vi "Execute.vi"(8 "error in":errorcluster, 11 "Wait STEP in":refnum<class "Wait STEP.lvclass">) -> (0 "error out":errorcluster, 1 "Next Step?":bool, 2 "MSG":string, 3 "Wait STEP out":refnum<class "Wait STEP.lvclass">)   [LabVIEW 2014, in "Wait STEP.lvclass"]
uses:
  Wait STEP.lvclass
  reusable/Sequence/STEPS/STEP.lvclass/STEP.ctl
  reusable/Sequence/STEPS/LEAVES/Double/Switch DBL.lvclass/Switch DBL.ctl
  reusable/Sequence/STEPS/Write First Call.vi
  reusable/Sequence/STEPS/Read First Call.vi
  reusable/Sequence/STEPS/LEAVES/Double/Read val.vi
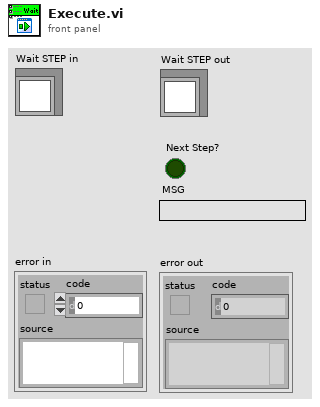
[diagram p1: front panel]
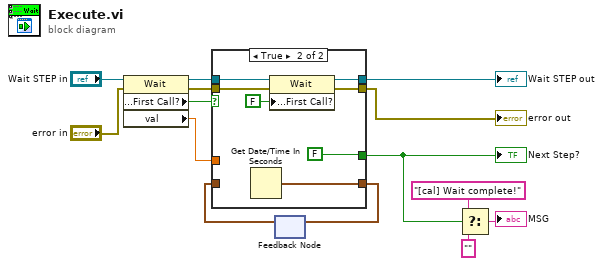
[diagram p0: block diagram]
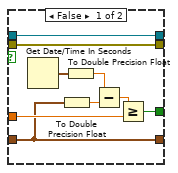
[diagram p2: hidden frame]
diagram:
  n1 = property class="Wait"(reference="Wait STEP in", error in="error in") -> (reference out=w12:refnum<class "Wait STEP.lvclass">, error out=w7:errorcluster, "Accessors:First Call?"=w13:bool, "val"=w10:dbl)
  n2 = feedback #1() -> (w11:timestamp)  [unwired: 1 in]
  n3 = case shown="True" w13 {
    tunnel: w12 -> [w20 w30]
    tunnel: [w16 w28] -> w1
    tunnel: w11 -> [w16 _]
    tunnel: w10 -> [w22 _]
    tunnel: [w21 FALSE] -> w5
    tunnel: [w20 w26] -> w9
    tunnel: w7 -> [w19 w25]
    tunnel: [w19 w24] -> w6
    frame False {
      n4 = Get Date/Time In Seconds() -> (seconds since 1Jan1904=w18:timestamp)
      n5 = To Double Precision Float(number=w16) -> (double precision float=w15:dbl)
      n6 = To Double Precision Float(number=w18) -> (double precision float=w17:dbl)
      n7 = Subtract(x=w17, y=w15) -> (x-y=w23:dbl)
      n8 = Greater Or Equal?(x=w23, y=w22) -> (x >= y?=w21:bool)
    }
    frame True {
      n9 = Get Date/Time In Seconds() -> (seconds since 1Jan1904=w28:timestamp)
      n10 = property class="Wait"(reference=w30, error in=w25, "Accessors:First Call?"=FALSE ("First Call?")) -> (reference out=w26:refnum<class "Wait STEP.lvclass">, error out=w24:errorcluster)
    }
  }
  "error out" <- w6
  "Wait STEP out" <- w9
  "Next Step?" <- w5
  n11 = feedback-in #1(w1) -> ()
  n12 = Select(t="[cal] Wait complete!", s=w5, f="") -> (s? t:f=→"MSG":string)
